vi "Init Fluidics.vi"(8 "error in (no error)":errorcluster, 11 "Application in":refnum<class "Application.lvclass">) -> (0 "error out":errorcluster, 3 "Application out":refnum<class "Application.lvclass">)   [LabVIEW 2023, in "Application.lvlib" / "Application.lvclass"]
uses:
  Application.lvclass
  C:/Program Files/National Instruments/LabVIEW 2023/vi.lib/ActorFramework/Actor/Actor.lvclass
  Application.lvclass/Application.ctl
  User Interface/Splash Screen Messages/Update Status Msg/Update Status Msg.lvclass/Update Status Msg.ctl
  <vilib>/ActorFramework/Message Enqueuer/Message Enqueuer.lvclass/Message Enqueuer.ctl
  <vilib>/ActorFramework/Message Enqueuer/Enqueue.vi
  User Interface/Splash Screen Messages/Update Status Msg/Update Status Msg.lvclass
  C:/Program Files/National Instruments/LabVIEW 2023/vi.lib/ActorFramework/Message/Message.lvclass
  Hardware/Autosampler/Autosampler.lvclass
  <vilib>/ActorFramework/Message Priority Queue/Priority Enqueue.vi
  <vilib>/ActorFramework/Actor/Actor.lvclass
  C:/FLASH/Development/Hardware/Device/Device.lvclass
  C:/FLASH/Development/Hardware/Autosampler/Autosampler.lvclass
  C:/FLASH/Development/Application/Application.lvclass
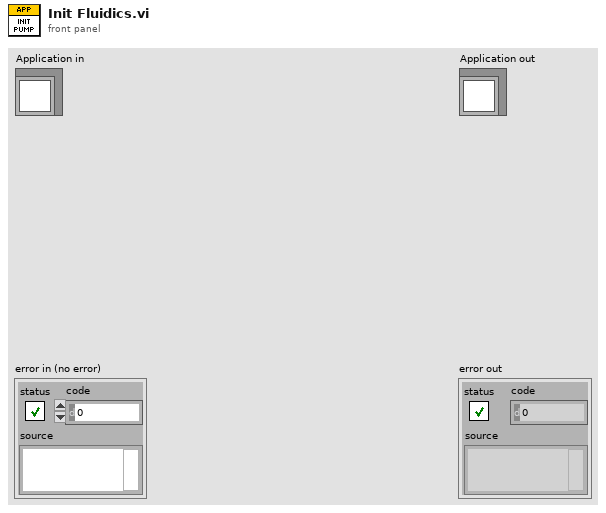
[diagram p1: front panel]
types:
  T1 = typedef "Autosampler Configuration.ctl" = cluster{"Serial Port":refnum<visa-resource-name>, "Device Type":enum16{"Disabled", "Simulate", "Alltesta"}}
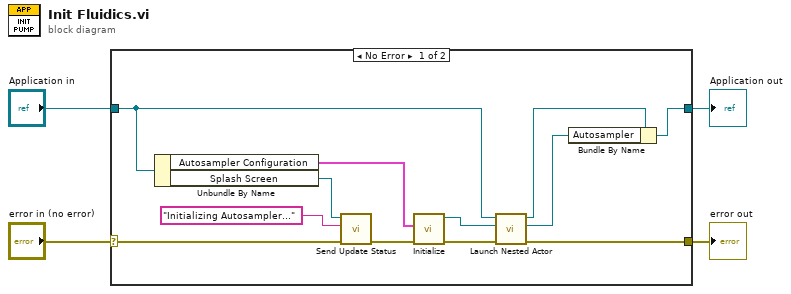
[diagram p0: block diagram]
diagram:
  n1 = case shown="No Error" "error in (no error)" {
    selector: "error in (no error)" -> [w16 w18]
    tunnel: [w12 w18] -> w3
    tunnel: [w11 w17] -> w1
    tunnel: "Application in" -> [w9 w17]
    frame No Error {
      n2 = Unbundle By Name(w9) -> ("Autosampler Configuration"=w5:T1, "Splash Screen"=w15:refnum<class "Message Enqueuer.lvclass">)
      n3 = call "Send Update Status.vi"("error in (no error)"=w16, "Status Message"="Initializing Autosampler...", "Message Enqueuer"=w15) -> ("error out"=w6:errorcluster)  [unwired: 7 in, 1 out]
      n4 = call "Initialize.vi"("error in (no error)"=w6, "Fluidics Configuration"=w5) -> ("error out"=w13:errorcluster, "Autosampler out"=w10:refnum<class "Autosampler.lvclass">)  [unwired: 8 in]
      n5 = call <vilib>:"Launch Nested Actor.vi"("error in (no error)"=w13, "Nested Actor"=w10, "Caller Actor in"=w9) -> ("error out"=w12:errorcluster, "Nested Actor's Enqueuer"=w7:refnum<class "Message Enqueuer.lvclass">, "Caller Actor out"=w8:refnum<class "Application.lvclass">)  [unwired: 6 in]
      n6 = Bundle By Name(cluster=w8, "Autosampler"=w7) -> (w11:refnum<class "Application.lvclass">)
    }
    frame Error {
    }
  }
  "error out" <- w3
  "Application out" <- w1
